vi "Peak averager.vi"(8 "Marker Freq stop":dbl, 9 "Marker Freq start":dbl, 10 "Input Ys":dbl[](array[numeric]), 11 "Input Xs":dbl[](array[numeric])) -> (1 "mean of peak":dbl format="%0.2f", 2 "Amp in range 2":dbl[](array[numeric]), 3 "Pts in range 2":dbl[](array[numeric]))   [LabVIEW 2016]
uses:
  <vilib>/Analysis/baseanly.llb/Mean (DBL).vi
  <vilib>/Analysis/NI_AALBase.lvlib
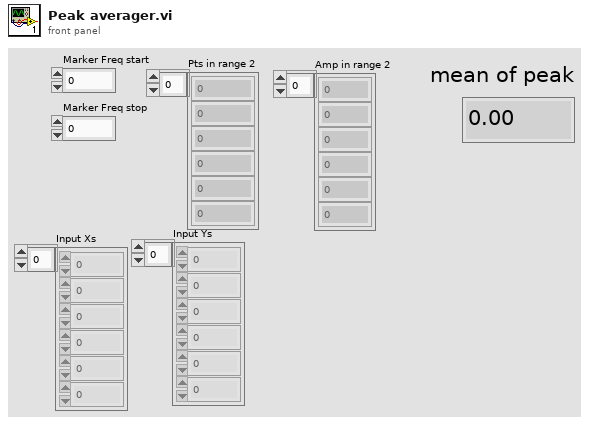
[diagram p1: front panel]
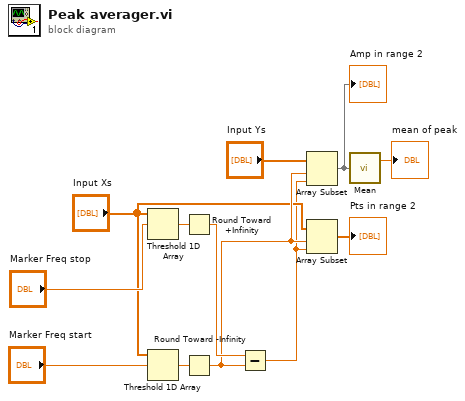
[diagram p0: block diagram]
diagram:
  n1 = Threshold 1D Array(2:"Marker Freq stop", 3:"Input Xs") -> (0:w10:dbl)  [unwired: 1 in]
  n2 = Threshold 1D Array(2:"Marker Freq start", 3:"Input Xs") -> (0:w9:dbl)  [unwired: 1 in]
  n3 = Round Toward +Infinity(x=w10) -> (ceil(x): smallest int >= x=w8:dbl)
  n4 = Round Toward -Infinity(1:w9) -> (0:w6:dbl)
  n5 = Subtract(x=w8, y=w6) -> (x-y=w1:dbl)
  n6 = Array Subset(array="Input Ys", index=w6, length=w1) -> (w4:dbl[])
  "Amp in range 2" <- w4
  n7 = Array Subset(array="Input Xs", index=w6, length=w1) -> (→"Pts in range 2":dbl[])
  n8 = call-poly <vilib>:"Mean.vi"("X"=w4) -> ("mean"=→"mean of peak":dbl)  [unwired: 1 out]
